vi "SEQ Obtain.vi"(8 "error in":errorcluster) -> (0 "error out":errorcluster, 3 "queue out":refnum<queue>)   [LabVIEW 2019, in "sbRIO9623.lvlib"]
uses:
  sbRIO9623.lvlib
  SEQ Data.ctl
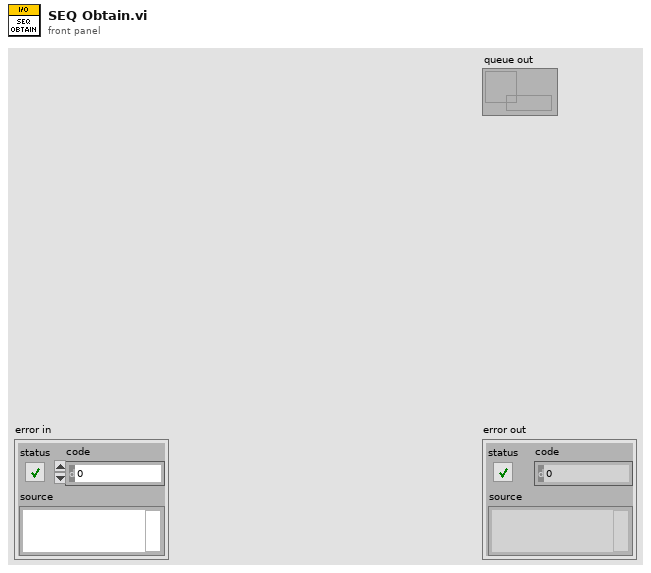
[diagram p1: front panel]
types:
  T1 = typedef "sbRIO9623.lvlib/SEQ Data.ctl" = cluster{"Lid Sensor 1":bool, "Lid Sensor 2":bool, "Laser Interlock":bool, "Buffer Tank":bool, "Wash Tank":bool, "Waste Tank":bool, "SiPM 1":fxp<+,20,5>, "SiPM 2":fxp<+,20,5>, "Initialize Success?":bool, "VI Refnum":refnum<vi>}
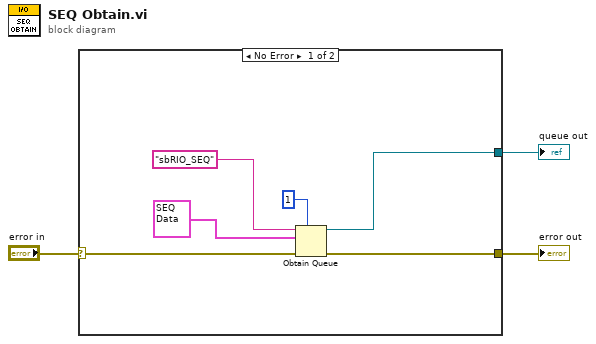
[diagram p0: block diagram]
diagram:
  n1 = case shown="No Error" "error in" {
    selector: "error in" -> [w9 w10]
    tunnel: [w8 w10] -> w2
    tunnel: [w4 _] -> w1
    frame No Error {
      n2 = Obtain Queue(max queue size (-1, unlimited)=1, name (unnamed)="sbRIO_SEQ", element data type=T1 {"Lid Sensor 1"=FALSE, "Lid Sensor 2"=FALSE, "Laser Interlock"=FALSE, "Buffer Tank"=FALSE, "Wash Tank"=FALSE, "Waste Tank"=FALSE, "SiPM 1"=0.0, "SiPM 2"=0.0, "Initialize Success?"=FALSE, "VI Refnum"=refnum} ("Cluster"), error in (no error)=w9) -> (queue out=w4:refnum<queue>, error out=w8:errorcluster)  [unwired: 1 in, 1 out]
    }
    frame Error {
    }
  }
  "error out" <- w2
  "queue out" <- w1
